vi "Untitled 8.vi"() -> ()   [LabVIEW 2015]
panel:
  out "Discriminante":dbl
  out "Discriminante < 0":bool
  out "Discriminante = 0":bool
  out "Discriminante > 0":bool
  in  "Número C":dbl
  in  "Número A":dbl
  in  "Número B":dbl
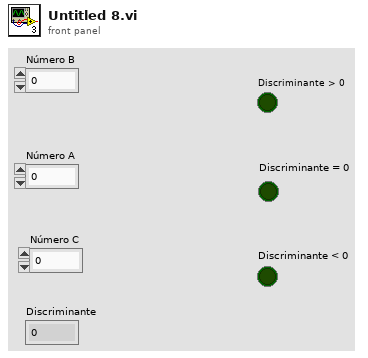
[diagram p1: front panel]
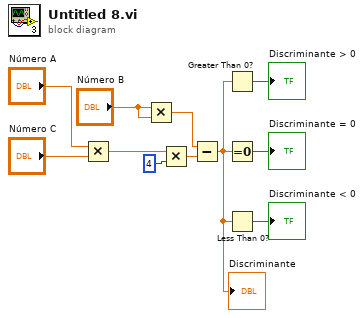
[diagram p0: block diagram]
diagram:
  n1 = Multiply(x="Número A", y="Número C") -> (x*y=w2:dbl)
  n2 = Multiply(x="Número B", y="Número B") -> (x*y=w10:dbl)
  n3 = Multiply(x=w2, y=4) -> (x*y=w1:dbl)
  n4 = Subtract(x=w10, y=w1) -> (x-y=w4:dbl)
  "Discriminante" <- w4
  n5 = Greater Than 0?(x=w4) -> (x > 0?=→"Discriminante > 0":bool)
  n6 = Equal To 0?(x=w4) -> (x = 0?=→"Discriminante = 0":bool)
  n7 = Less Than 0?(x=w4) -> (x < 0?=→"Discriminante < 0":bool)
